vi "Ballard XML Generator.HW Instructions.vi"(11 "string in":string) -> (3 "string out":string)   [LabVIEW 2020]
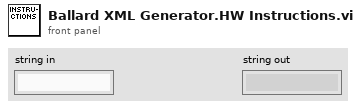
[diagram p1: front panel]
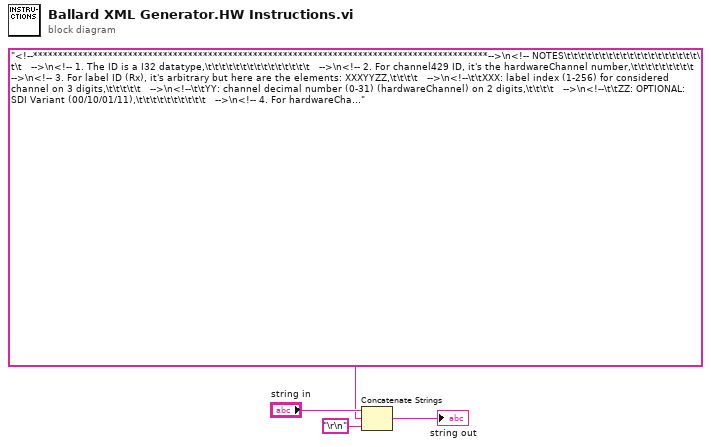
[diagram p0: block diagram]
diagram:
  n1 = Concatenate Strings("string in", "<!--*******************************************************************************************-->\n<!-- NOTES\t\t\t\t\t\t\t\t\t\t\t\t\t\t\t\t\t\t\t\t\t   -->\n<!-- 1. The ID is a I32 datatype,\t\t\t\t\t\t\t\t\t\t\t\t\t\t\t   -->\n<!-- 2. For channel429 ID, it's the hardwareChannel number,\t\t\t\t\t\t\t\t\t   -->\n<!-- 3. For label ID (Rx), it's arbitrary but here are the elements: XXXYYZZ,\t\t\t\t   -->\n<!--\t\tXXX: label index (1-256) for considered channel on 3 digits,\t\t\t\t\t   -->\n<!--\t\tYY: channel decimal number (0-31) (hardwareChannel) on 2 digits,\t\t\t\t   -->\n<!--\t\tZZ: OPTIONAL: SDI Variant (00/10/01/11),\t\t\t\t\t\t\t\t\t\t   -->\n<!-- 4. For hardwareChannel numbering, for a core with 16 (Rx/Tx) Channels, Rx Channels are\t   -->\n<!-- numbered between 0 and 15, Tx Channels are numbered between 16 and 31. Physically, for    -->\n<!-- instance, hardwareChannel 1 and 17 are the same but the direction is different.\t\t   -->\n<!-- 5. For message ID (Tx), it's arbitrary but here are the elements: XXXYYZZZ,\t\t\t   -->\n<!--\t\tXXX`: label index (1-256) for considered channel on 3 digits,\t\t\t\t\t   -->\n<!--\t\tYY: channel decimal number (0-31) (hardwareChannel) on 2 digits,\t\t\t\t   -->\n<!-- 6. For messageBuffer ID (Tx), it's arbitrary but here are the elements: XXXYYZZZ,\t\t   -->\n<!--\t\tXXX`: label index (1-999) for considered channel on 3 digits,\t\t\t\t\t   -->\n<!--\t\tYY: channel decimal number (0-31) (hardwareChannel) on 2 digits,\t\t\t\t   -->\n<!--\t\tZZZ: messageBuffer Index on 3 digits (1-999),\t\t\t\t\t\t\t\t\t   -->\n<!-- 7. For Rx Channels, it's important to list ALL labels physically present on the Channel   -->\n<!--    and, for each, set \"monitor\" element to true or false.\t\t\t\t\t\t\t\t   -->\n<!--*******************************************************************************************-->", "\r\n") -> (→"string out":string)
